vi "asdk Init.vi"(8 "error in (no error)":errorcluster, 11 "serialName":string) -> (0 "error out":errorcluster, 3 "function return":u64)   [LabVIEW 2017, in "ASDK.lvlib"]
doc: "ASDK_API asdkDM * asdkInit( CStrConst serialName );"
uses:
  ASDK.lvlib
  ASDK.dll
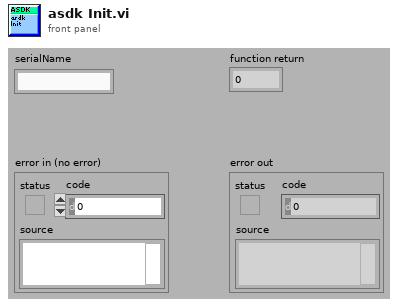
[diagram p1: front panel]
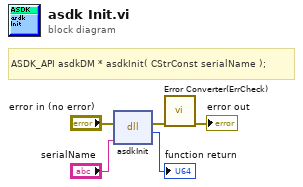
[diagram p0: block diagram]
diagram:
  # "ASDK_API asdkDM * asdkInit( CStrConst serialName );"
  n1 = dll-call lib="ASDK.*" fn="asdkInit"(error in="error in (no error)", "serialName"="serialName") -> (error out=w2:errorcluster, "return type"=→"function return":u64)  [unwired: 3 in, 1 out]
  n2 = call "Error Converter(ErrCheck).vi"("error in (no error)"=w2) -> ("error out"=→"error out":errorcluster)  [unwired: 10 in]
